vi "Get Buffers.vi"(11 "Framework in":refnum<class "Framework.lvclass">) -> (2 "Buffers":refnum<class "Buffers.lvclass">, 3 "Framework out":refnum<class "Framework.lvclass">)   [LabVIEW 2017, in "DSF Core.lvlib" / "Framework.lvclass"]
uses:
  Framework.lvclass
  Buffers/Buffers.lvclass
  Framework.lvclass/Framework.ctl
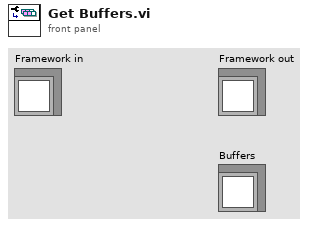
[diagram p1: front panel]
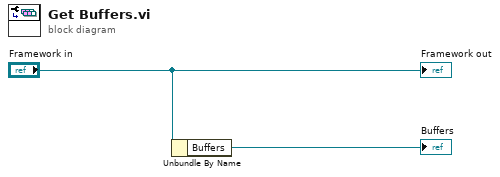
[diagram p0: block diagram]
diagram:
  n1 = Unbundle By Name("Framework in") -> ("Buffers"=→"Buffers":refnum<class "Buffers.lvclass">)
  "Framework out" <- "Framework in"
